vi "ExFlatAsyncExample.vi"() -> ()   [LabVIEW 2010]
panel:
  in  "Exposure":dbl format="%.2f"
  in  "stop":bool
  in  "Store":bool
  out "error out":errorcluster
  in  "error in (no error)":errorcluster
  # "ExFlatAsyncExample:\nThis example first takes one image for a flat field, \nthen collects continoously in async mode using \nthe first frame collected as the flat field frame."
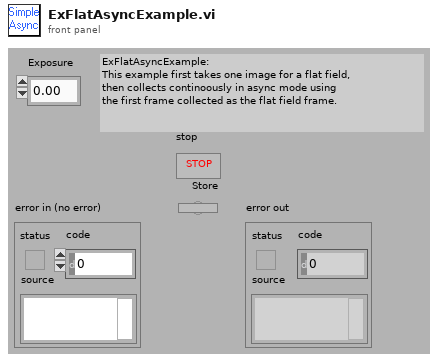
[diagram p1: front panel]
types:
  T1 = cluster{i32, "Xdim":u32, i32, i32, "Ydim":u32, i32}
  T2 = cluster{"Acquire Mode \n3-Async":i32, "Exposure":dbl, "Number of Images":i32, "Software accumulation":i32}
  T3 = cluster{"Camera Handle":u32, "Pulser Handle":u32, "File Handle":u32, "Display Handle":u32, "Image Handle":u32}
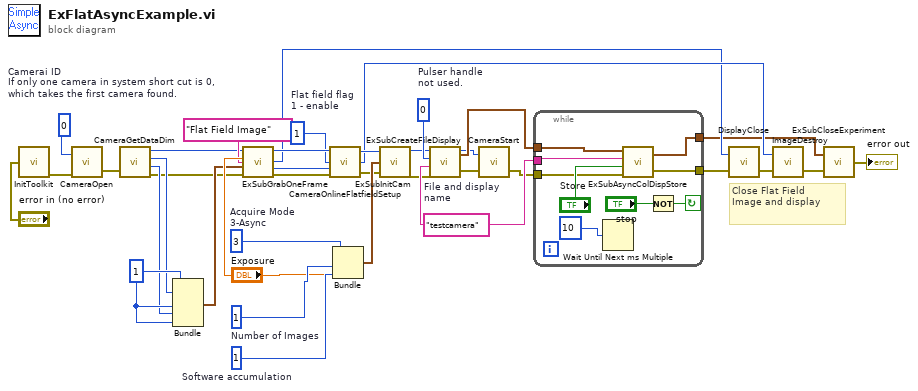
[diagram p0: block diagram]
diagram:
  w15 = 1
  w17 = 1  # Flat field flag 1 - enable
  w22 = 0  # Camerai ID If only one camera in system short cut is 0,  which takes the first camera found.
  w29 = 0  # Pulser handle not used.
  w34 = 1  # Number of Images
  w35 = 3  # Acquire Mode  3-Async
  w33 = 1  # Software accumulation
  w36 = "testcamera"  # File and display name
  # "Close Flat Field\nImage and display"
  n1 = call <userlib>:"InitToolkit.vi"("error in"="error in (no error)") -> ("error out"=w23:errorcluster)
  n2 = call <userlib>:"CameraOpen.vi"("error in"=w23, "Camera Device ID"=w22) -> ("error out"=w13:errorcluster)  [unwired: 1 out]
  n3 = call <userlib>:"CameraGetDataDim.vi"("error in"=w13) -> ("Camera Handle"=w4:u32, "Xdim"=w3:u32, "Ydim"=w2:u32, "error out"=w1:errorcluster)  [unwired: 1 in]
  n4 = Bundle(w15, "Xdim"=w3, w15, w15, "Ydim"=w2, w15) -> (w14:T1)  [unwired: 1 in]
  n5 = call "ExSubGrabOneFrame.vi"("Display Title"="Flat Field Image", "error in"=w1, "ROI Cluster"=w14, "Exposure"="Exposure", "Camera Handle"=w4) -> ("error out"=w16:errorcluster, "Image Handle"=w18:u32, "Display Handle"=w10:u32, "Camera Handle out"=w19:u32)
  n6 = call <userlib>:"CameraOnlineFlatfieldSetup.vi"("error in"=w16, "Flat Field Flag"=w17, "Flat Field Image Handle"=w18, "Camera Handle"=w19) -> ("error out"=w20:errorcluster, "Flat Field Image Handle"=w11:u32, "Camera Handle"=w21:u32)
  n7 = Bundle("Acquire Mode \n3-Async"=w35, "Exposure"="Exposure", "Number of Images"=w34, "Software accumulation"=w33) -> (w31:T2)  [unwired: 1 in]
  n8 = call "ExSubInitCam.vi"("error in (no error)"=w20, "Camera Information"=w31, "Camera Handle"=w21) -> ("error out"=w30:errorcluster, "Camera Handle"=w25:u32)
  n9 = call "ExSubCreateFileDisplay.vi"("error in (no error)"=w30, "File and Display Name"=w36, "Pulser Handle"=w29, "Camera Handle"=w25) -> ("error out"=w28:errorcluster, "Handles Out"=w27:T3)
  n10 = call <userlib>:"CameraStart.vi"("error in"=w28, "Camera Handle"=w25) -> ("error out"=w26:errorcluster)  [unwired: 1 out]
  n11 = while {
    tunnel: w27 -> [w43]
    tunnel: w26 -> [w41]
    tunnel: w36 -> [w42]
    tunnel: [w39] -> w8
    tunnel: [w40] -> w7
    stop <- w38 continue-if-true
    n12 = Wait Until Next ms Multiple(millisecond multiple=10) -> ()  [unwired: 1 out]
    n13 = call "ExSubAsyncColDispStore.vi"("error in (no error)"=w41, "Store Data"="Store", "Display Title"=w42, "Handle Cluster"=w43) -> ("error out"=w39:errorcluster, "Handle Cluster Out"=w40:T3)
    n14 = Not(x="stop") -> (.not. x?=w38:bool)
  }
  n15 = call <userlib>:"DisplayClose.vi"("error in"=w8, "Display Handle"=w10) -> ("error out"=w9:errorcluster)
  n16 = call <userlib>:"ImageDestroy.vi"("error in"=w9, "Data handle"=w11) -> ("error out"=w6:errorcluster)
  n17 = call "ExSubCloseExperiment.vi"("error in (no error)"=w6, "Handles In"=w7) -> ("error out"=→"error out":errorcluster)
